vi "comm get cts.vi"(8 "error in (no error)":errorcluster, 11 "Comm Handle":u32) -> (0 "error out":errorcluster, 2 "CTS":bool, 3 "dup Comm Handle":u32)   [LabVIEW 2017, in "lvserial.lvlib"]
doc: "Retrieves modem control-register values."
uses:
  lvserial.lvlib
  lvserial.dll
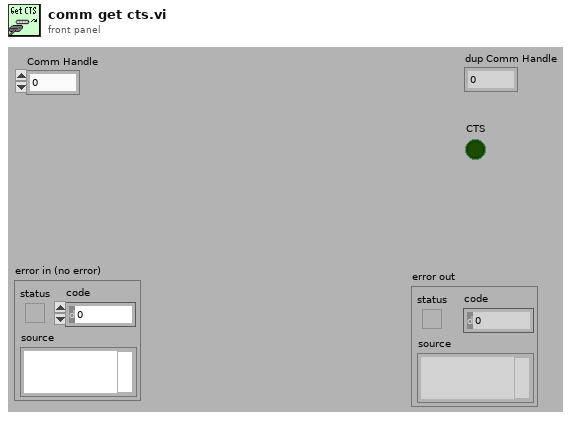
[diagram p1: front panel]
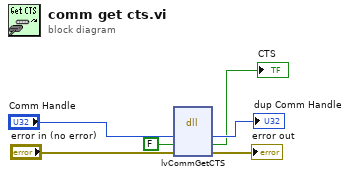
[diagram p0: block diagram]
diagram:
  n1 = dll-call lib="lvserial.dll" fn="lvCommGetCTS"("hComm"="Comm Handle", "CTS"=FALSE, "error in (no error)"="error in (no error)") -> ("hComm"=→"dup Comm Handle":u32, "CTS"=→"CTS":bool, "error in (no error)"=→"error out":errorcluster)  [unwired: 3 in, 3 out]
